vi "颜色识别.vi"(2 "Exit Event":refnum<user-event>) -> ()   [LabVIEW 2018]
uses:
  <vilib>/userdefined/High Color/IMAQdx.ctl
  <vilib>/vision/Image Controls.llb/IMAQ Image.ctl
  <vilib>/vision/driver/IMAQdx.llb/IMAQdx Acquisition Mode.ctl
  <vilib>/vision/NI_Vision_Development_Module.lvlib
  <vilib>/vision/driver/NI_Vision_Acquisition_Software.lvlib
panel:
  in  "识别":bool
  in  "Rectangle":T1 {"Rotation" min=-90.0 max=90.0 step=1.0 format="%.2f"}
  in  "IMAQdx Session":T2
  in  "stop":bool
  in  "开始":bool
  in  "静态/实时":bool
  out "Yellow":bool
  out "Green":bool
  out "Red":bool
  out "Color Spectrum":dbl[](array[numeric]) format="%.2f"
  out "Image":T3(plugin-control)
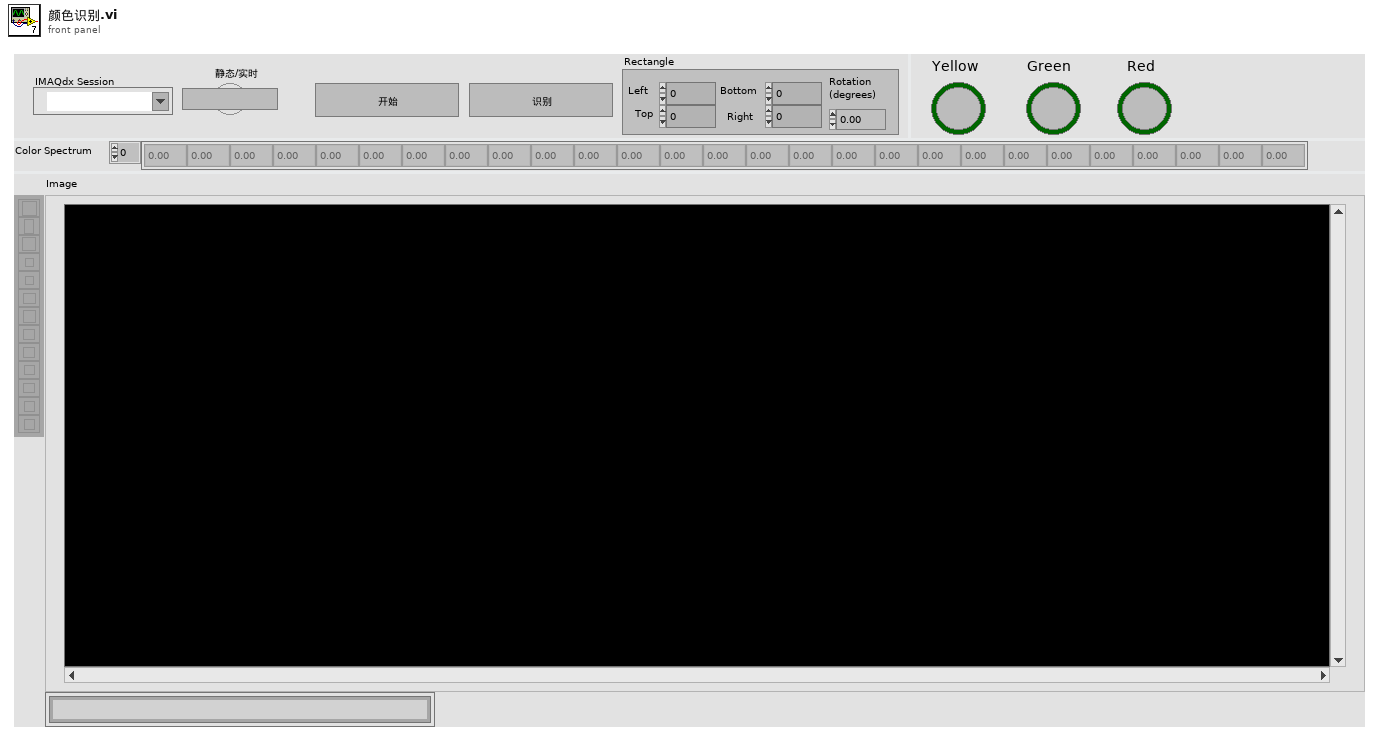
[diagram p1: front panel]
types:
  T1 = cluster{"Left":i32, "Top":i32, "Right":i32, "Bottom":i32, "Rotation":dbl}
  T2 = typedef "IMAQdx.ctl" = refnum<k21>
  T3 = typedef "IMAQ Image.ctl" = refnum<image>
  T4 = enum8{"Enabled", "Disabled", "Disabled and Grayed Out"}
  T5 = typedef "NI_Vision_Acquisition_Software.lvlib/IMAQdx Acquisition Mode.ctl" = enum32{"One Shot", "Continuous"}
  T6 = typedef "Image Type" = u32
  T7 = typedef "ROI Descriptor" = cluster{"Global Rectangle":i32[], "Contours":cluster{"ID":enum32{"External", "Internal"}, "Type":u32, "Coordinates":i32[]}[]}
  T8 = cluster{"Global Rectangle":i32[], "Contours":cluster{"Contour Type":u32, "ROI Type":u32, "Points":i32[]}[]}
  T9 = typedef "IMAQ Rectangle" = cluster{"Left":i32, "Top":i32, "Right":i32, "Bottom":i32, "Rotation":dbl}
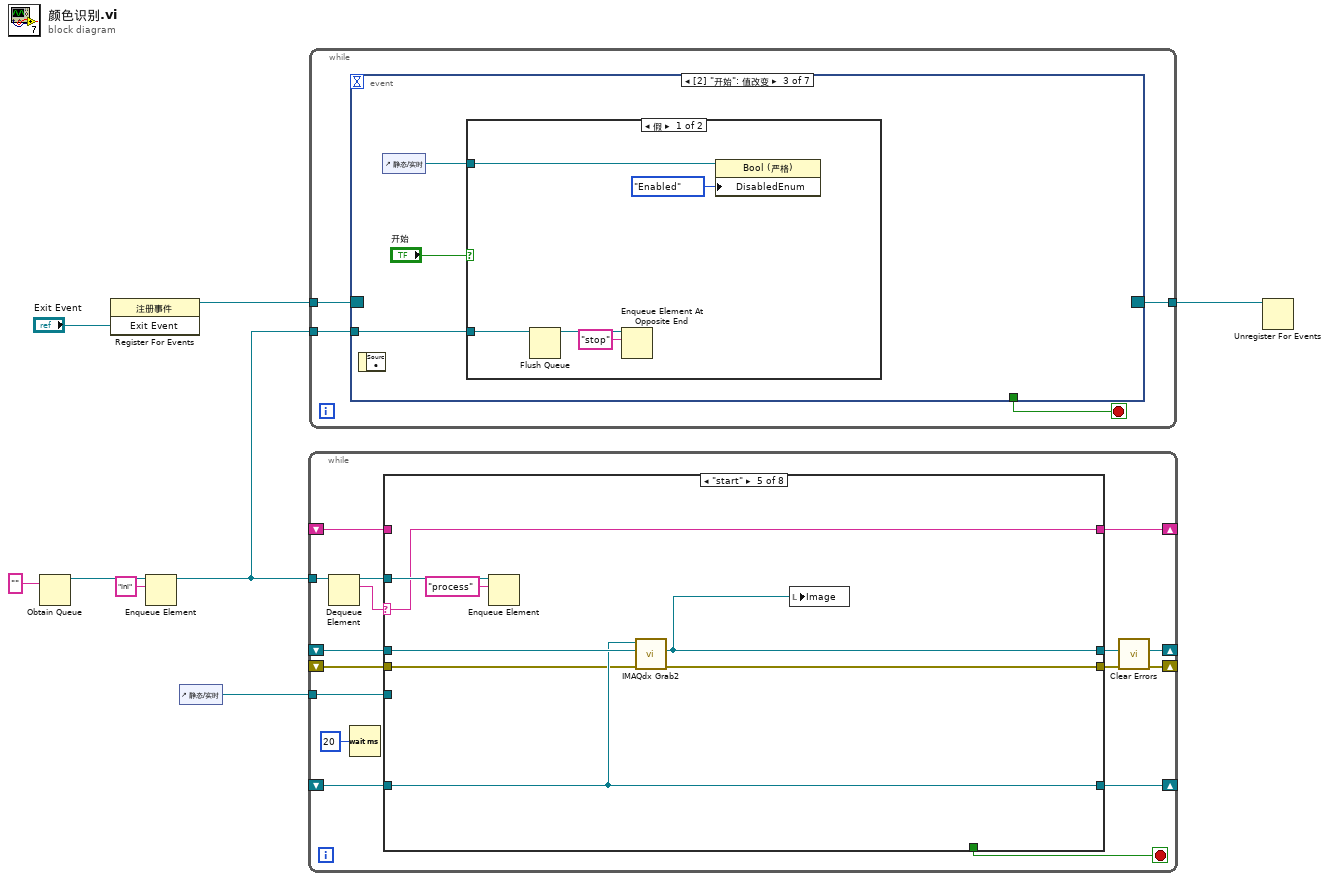
[diagram p0: block diagram]
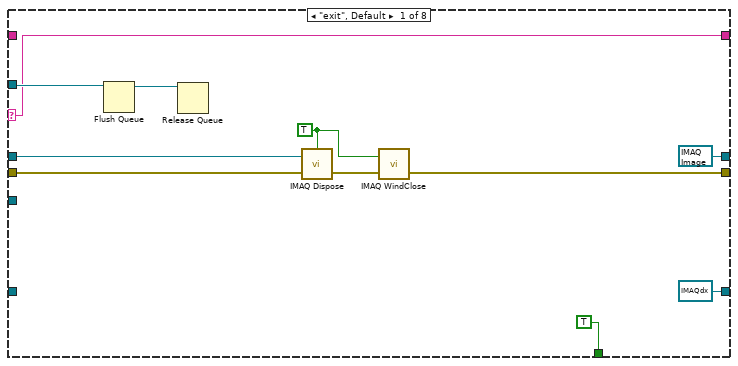
[diagram p2: hidden frame]
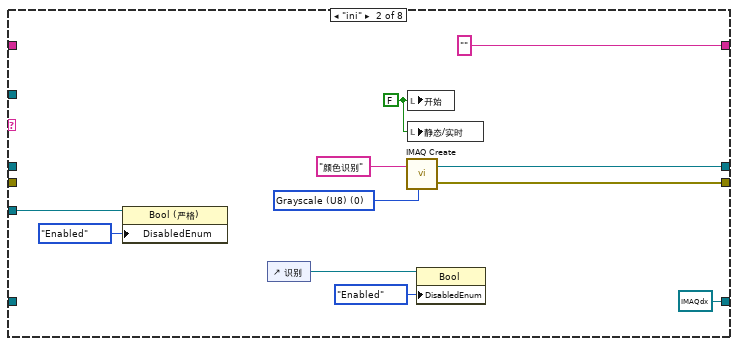
[diagram p3: hidden frame]
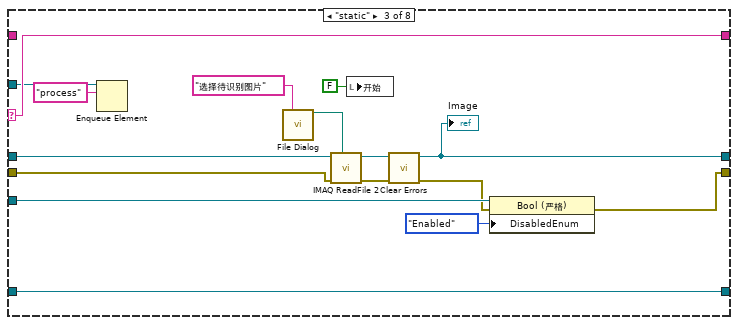
[diagram p4: hidden frame]
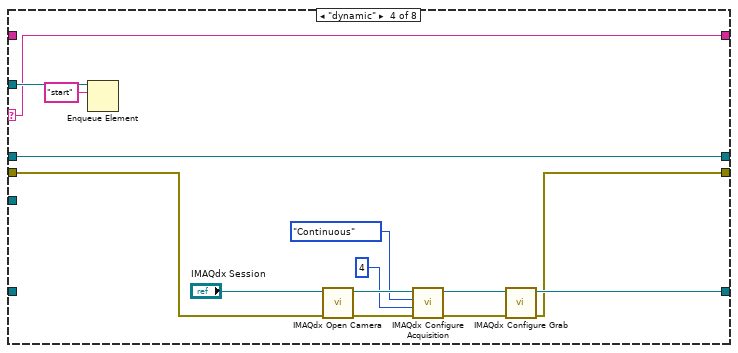
[diagram p5: hidden frame]
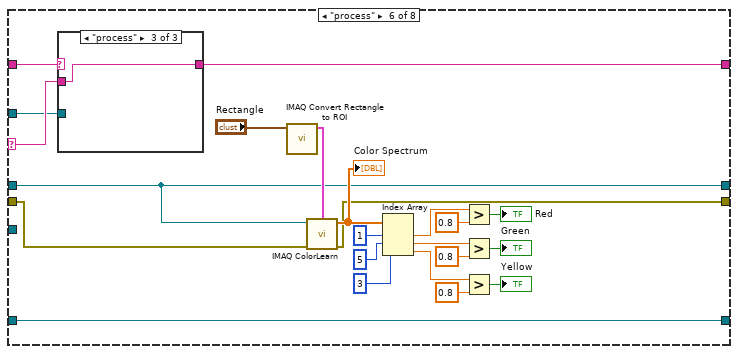
[diagram p6: hidden frame]
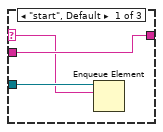
[diagram p7: hidden frame]
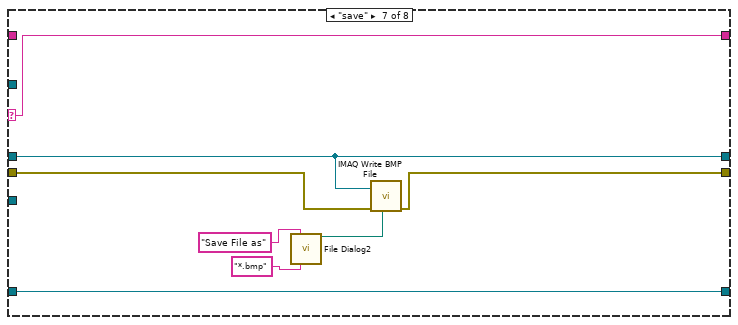
[diagram p9: hidden frame]
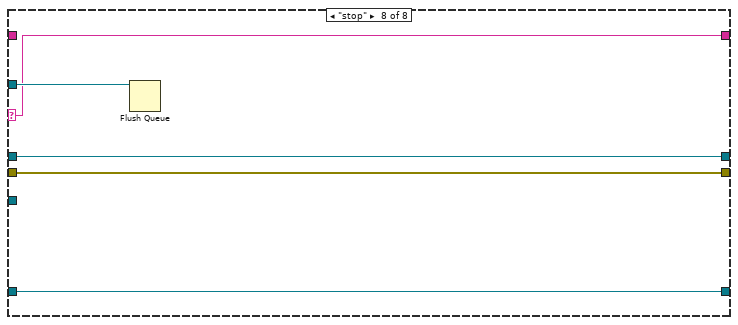
[diagram p10: hidden frame]
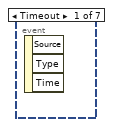
[diagram p11: hidden frame]
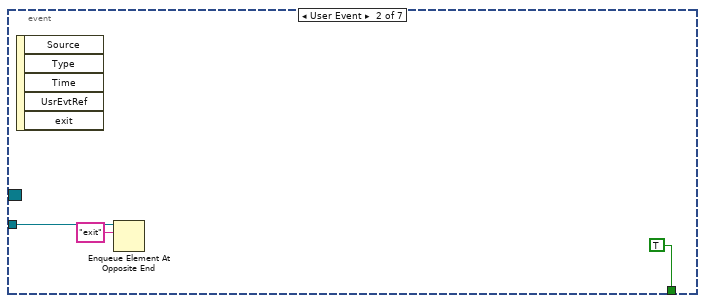
[diagram p12: hidden frame]
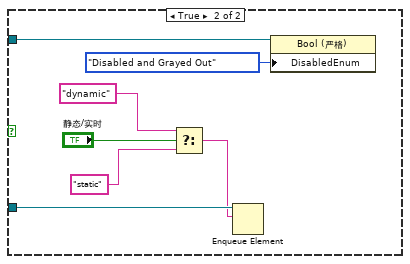
[diagram p13: hidden frame]
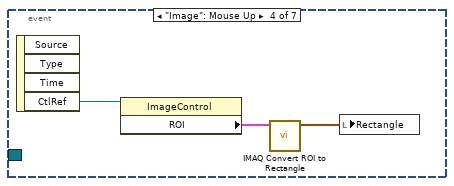
[diagram p14: hidden frame]
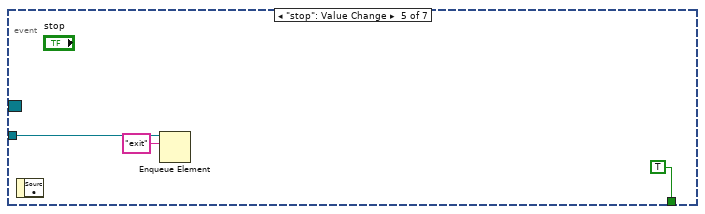
[diagram p15: hidden frame]
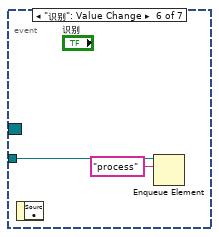
[diagram p16: hidden frame]
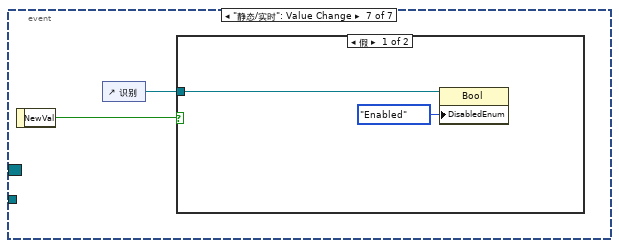
[diagram p17: hidden frame]
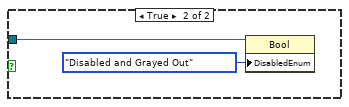
[diagram p18: hidden frame]
diagram:
  n1 = Obtain Queue(element data type="") -> (queue out=w5:refnum<queue>)  [unwired: 4 in, 2 out]
  n2 = register-events("Exit Event") -> (reference out=w2:refnum<event-registration>)  [unwired: 2 in, 1 out]
  n3 = Enqueue Element(queue=w5, element="ini") -> (queue out=w3:refnum<queue>)  [unwired: 2 in, 2 out]
  n4 = control-ref of="静态/实时"() -> (w1:refnum<vi>)
  n5 = while {
    tunnel: w3 -> [w23]
    shift-right: [w19] -> _
    shift-left: _ -> [w18]
    shift-right: [w17] -> _
    shift-left: _ -> [w16]
    shift-right: [w15] -> _
    shift-left: _ -> [w14]
    tunnel: w1 -> [w13]
    shift-right: [w10] -> _
    shift-left: _ -> [w11]
    stop <- w20 stop-if-true
    n6 = Dequeue Element(queue=w23) -> (queue out=w21:refnum<queue>, element=w22:string)  [unwired: 2 in, 2 out]
    n7 = Wait (ms)(milliseconds to wait=u32 20 ("等待时间（毫秒）")) -> ()  [unwired: 1 out]
    n8 = case shown="\"start\"" w22 {
      selector: w22 -> [w26 _ w58 w69 w79 w103 w113 w120]
      tunnel: w21 -> [w34 _ w57 w71 w80 w101 _ w123]
      tunnel: [TRUE _ _ _ _ _ _ _] -> w20
      tunnel: [T3 refnum ("New Image") w41 w53 w72 w75 w86 w115 w122] -> w19
      tunnel: w18 -> [w29 _ w52 w72 w82 w86 w115 w122]
      tunnel: [T2 refnum ("Session Out") T2 refnum ("Session Out") w59 w64 w81 w105 w114 w121] -> w17
      tunnel: w16 -> [_ _ w59 _ w81 w105 w114 w121]
      tunnel: [w26 "" w58 w69 w79 w102 w113 w120] -> w15
      tunnel: w14 -> [_ _ _ _ _ w104 _ _]
      tunnel: w13 -> [_ w36 w50 _ _ _ _ _]
      tunnel: [w25 w35 w48 w62 w76 w83 w111 w119] -> w12
      tunnel: w11 -> [w24 _ w46 w68 w77 w84 w112 w119]
      frame "exit", Default {
        w30 = TRUE ("All Images? (No)")
        n9 = Flush Queue(queue=w34) -> (queue out=w33:refnum<queue>)  [unwired: 1 in, 2 out]
        n10 = Release Queue(queue=w33) -> ()  [unwired: 2 in, 3 out]
        n11 = call "IMAQ Dispose"("All Images? (No)"=w30, "Image"=w29, "error in (no error)"=w24) -> ("error out"=w31:errorcluster)  [unwired: 3 in]
        n12 = call "IMAQ WindClose"("Close All Windows (False)"=w30, "error in (no error)"=w31) -> ("error out"=w25:errorcluster)  [unwired: 4 in]
      }
      frame "ini" {
        w38 = FALSE ("开始")
        w42 = T6 0 items=["Grayscale (U8)", "Grayscale (I16)", "Grayscale (SGL)", "Complex (CSG)", "RGB (U32)", "HSL (U32)", "RGB (U64)", "Grayscale (U16)"] ("Image Type")
        n13 = property class="Bool (严格)"(reference=w36, "DisabledEnum"=T4."Enabled" ("Disabled")) -> ()  [unwired: 1 in, 2 out]
        n14 = control-ref of="识别"() -> (w39:refnum<vi>)
        n15 = call "IMAQ Create"("Image Name"="颜色识别", "Image Type"=w42) -> ("New Image"=w41:T3, "error out"=w35:errorcluster)  [unwired: 3 in]
        n16 = local write "开始"(w38) -> ()
        n17 = local write "静态/实时"(w38) -> ()
        n18 = property class="Bool"(reference=w39, "DisabledEnum"=T4."Enabled" ("Disabled")) -> ()  [unwired: 1 in, 2 out]
      }
      frame "static" {
        n19 = Enqueue Element(queue=w57, element="process") -> ()  [unwired: 2 in, 3 out]
        n20 = call "File Dialog"("prompt"="选择待识别图片") -> ("selected path"=w54:path)  [unwired: 11 in, 3 out]
        n21 = call "IMAQ ReadFile 2"("File Path"=w54, "error in (no error)"=w46, "Image"=w52) -> ("error out"=w49:errorcluster, "Image Out"=w53:T3)  [unwired: 4 in, 3 out]
        "Image" <- w53
        n22 = local write "开始"(FALSE ("开始")) -> ()
        n23 = call <vilib>:"Clear Errors.vi"("error in (no error)"=w49) -> ("error out"=w47:errorcluster)  [unwired: 5 in, 1 out]
        n24 = property class="Bool (严格)"(reference=w50, error in=w47, "DisabledEnum"=T4."Enabled" ("Disabled")) -> (error out=w48:errorcluster)  [unwired: 1 out]
      }
      frame "dynamic" {
        n25 = Enqueue Element(queue=w71, element="start") -> ()  [unwired: 2 in, 3 out]
        n26 = call <vilib>:"IMAQdx Open Camera.vi"("error in"=w68, "Session In"="IMAQdx Session") -> ("error out"=w61:errorcluster, "Session Out"=w74:T2)  [unwired: 8 in]
        n27 = call <vilib>:"IMAQdx Configure Acquisition.vi"("error in"=w61, "Number of Buffers"=u32 4, "Continuous?"=IMAQdx_Acquisition_Mode."Continuous", "Session In"=w74) -> ("error out"=w63:errorcluster, "Session Out"=w65:T2)  [unwired: 6 in]
        n28 = call <vilib>:"IMAQdx Configure Grab.vi"("error in"=w63, "Session In"=w65) -> ("error out"=w62:errorcluster, "Session Out"=w64:T2)  [unwired: 8 in]
      }
      frame "start" {
        n29 = Enqueue Element(queue=w80, element="process") -> ()  [unwired: 2 in, 3 out]
        n30 = call <vilib>:"IMAQdx Grab2.vi"("error in"=w77, "Image In"=w82, "Session In"=w81) -> ("error out"=w76:errorcluster, "Image Out"=w75:T3)  [unwired: 5 in, 2 out]
        n31 = local write "Image"(w75) -> ()
      }
      frame "process" {
        n32 = case shown="\"process\"" w104 {
          selector: w104 -> [w106 _ _]
          tunnel: w103 -> [w107 w109 w110]
          tunnel: [w107 w109 w110] -> w102
          tunnel: w101 -> [w108 _ _]
          frame "start", Default {
            n33 = Enqueue Element(queue=w108, element=w106) -> ()  [unwired: 2 in, 3 out]
          }
          frame "static" {
          }
          frame "process" {
          }
        }
        n34 = call "IMAQ Convert Rectangle to ROI"("Rectangle"="Rectangle") -> ("ROI Descriptor"=w93:T7)  [unwired: 8 in, 1 out]
        n35 = call "IMAQ ColorLearn"("ROI Descriptor"=w93, "Image"=w86, "error in (no error)"=w84) -> ("Color Spectrum"=w94:dbl[], "error out"=w83:errorcluster)  [unwired: 5 in]
        "Color Spectrum" <- w94
        n36 = Index Array(array=w94, index #1=1 ("索引"), index #2=5 ("索引"), index #3=3 ("索引")) -> (element #1=w95:dbl, element #2=w98:dbl, element #3=w100:dbl)
        n37 = Greater?(x=w95, y=0.8) -> (0:→"Red":bool)
        n38 = Greater?(x=w98, y=0.8) -> (0:→"Green":bool)
        n39 = Greater?(x=w100, y=0.8) -> (0:→"Yellow":bool)
      }
      frame "save" {
        n40 = call "File Dialog2"("prompt"="Save File as", "pattern (all files)"="*.bmp" ("pattern")) -> ("selected path"=w118:path)  [unwired: 10 in, 3 out]
        n41 = call "IMAQ Write BMP File"("error in (no error)"=w112, "File Path"=w118, "Image"=w115) -> ("error out"=w111:errorcluster)  [unwired: 5 in]
      }
      frame "stop" {
        n42 = Flush Queue(queue=w123) -> ()  [unwired: 1 in, 3 out]
      }
    }
    n43 = call <vilib>:"Clear Errors.vi"("error in (no error)"=w12) -> ("error out"=w10:errorcluster)  [unwired: 5 in, 1 out]
  }
  n44 = while {
    tunnel: w2 -> [w127]
    tunnel: [w126] -> w7
    tunnel: w3 -> [w124]
    stop <- w125 stop-if-true
    n45 = event shown="[2] \"开始\": 值改变" {
      selector: w127 -> [_ _ _ _ _ _ _]
      dyn-events: [_ _ _ _ _ _ _] -> w126
      timeout: _ -> [_ _ _ _ _ _ _]
      tunnel: [_ TRUE _ _ TRUE _ _] -> w125
      tunnel: w124 -> [_ w129 w133 _ w150 w153 _]
      event Timeout {
        n46 = event-data() -> ()  [unwired: 1 in, 3 out]
      }
      event User Event {
        n47 = event-data() -> ()  [unwired: 1 in, 5 out]
        n48 = Enqueue Element At Opposite End(queue=w129, element="exit") -> ()  [unwired: 2 in, 3 out]
      }
      event "开始": Value Change {
        n49 = event-data() -> ()  [unwired: 1 in, 1 out]
        n50 = control-ref of="静态/实时"() -> (w131:refnum<vi>)
        n51 = case shown="假" "开始" {
          tunnel: w133 -> [w138 w145]
          tunnel: w131 -> [w135 w140]
          frame False {
            n52 = Flush Queue(queue=w138) -> (queue out=w137:refnum<queue>)  [unwired: 1 in, 2 out]
            n53 = Enqueue Element At Opposite End(queue=w137, element="stop") -> ()  [unwired: 2 in, 3 out]
            n54 = property class="Bool (严格)"(reference=w135, "DisabledEnum"=T4."Enabled" ("Disabled")) -> ()  [unwired: 1 in, 2 out]
          }
          frame True {
            n55 = Select(t="dynamic" ("f"), s="静态/实时", f="static" ("element")) -> (s? t:f=w143:string)
            n56 = Enqueue Element(queue=w145, element=w143) -> ()  [unwired: 2 in, 3 out]
            n57 = property class="Bool (严格)"(reference=w140, "DisabledEnum"=T4."Disabled and Grayed Out" ("Disabled")) -> ()  [unwired: 1 in, 2 out]
          }
        }
      }
      event "Image": Mouse Up {
        n58 = event-data() -> ("CtlRef"=w146:refnum<vi>)  [unwired: 1 in, 3 out]
        n59 = property class="ImageControl"(reference=w146) -> ("ROI"=w148:T8)  [unwired: 1 in, 2 out]
        n60 = call "IMAQ Convert ROI to Rectangle"("ROI Descriptor"=w148) -> ("Rectangle"=w147:T9)  [unwired: 8 in, 1 out]
        n61 = local write "Rectangle"(w147) -> ()
      }
      event "stop": Value Change {
        n62 = event-data() -> ()  [unwired: 1 in, 1 out]
        n63 = Enqueue Element(queue=w150, element="exit") -> ()  [unwired: 2 in, 3 out]
      }
      event "识别": Value Change {
        n64 = event-data() -> ()  [unwired: 1 in, 1 out]
        n65 = Enqueue Element(queue=w153, element="process") -> ()  [unwired: 2 in, 3 out]
      }
      event "静态/实时": Value Change {
        n66 = event-data() -> ("NewVal"=w155:bool)  [unwired: 1 in]
        n67 = control-ref of="识别"() -> (w154:refnum<vi>)
        n68 = case shown="假" w155 {
          tunnel: w154 -> [w156 w159]
          frame False {
            n69 = property class="Bool"(reference=w156, "DisabledEnum"=T4."Enabled" ("Disabled")) -> ()  [unwired: 1 in, 2 out]
          }
          frame True {
            n70 = property class="Bool"(reference=w159, "DisabledEnum"=T4."Disabled and Grayed Out" ("Disabled")) -> ()  [unwired: 1 in, 2 out]
          }
        }
      }
    }
  }
  n71 = Unregister For Events(event registration refnum=w7) -> ()  [unwired: 1 in, 1 out]
